vi "Vision Research Phantom Series PhFile PhGetOpenCineName.vi"(4 "Options":u32(ring) items=["0", "OFN_MULTISELECT"], 5 "Error In (no error)":errorcluster) -> (15 "szFileName":path, 18 "Success":bool, 19 "Error Out":errorcluster)   [LabVIEW 2013, in "VRI.lvlib"]
doc: "PhFile.dll\n\nPhGetOpenCineName\nBOOL PhGetOpenCineName(PSTR szFileName, UINT Options);\n\nParameters Description\nszFileName (out) Name of the file selected from the dialog box.\nOptions(in) Options available:\n 0 – The user can select only one file name.\n OFN_MULTISELECT – The user can select one or more file names.\nReturn TRUE - The operation has succeeded. The user ended the dialog with OK.\n FALSE - The operation has been canceled. The user ended the dialog with CANCEL.\nComments This function displays a dialog box, for selecting one existing cine file.\n The file name is returned in the parameter.\n\nWritten by:\nBLOOMY CONTROLS, INC\nWINDSOR, CT 06095, USA\n860-298-9925\nwww.bloomy.com\nV1.0.0\nMay, 2004"
uses:
  VRI.lvlib
  Phantom DLLs/PhFile.dll
panel:
  # "For instructions on the use of this VI, press Ctrl+H to display the help window and move the mouse over the icon, controls, and indicators"
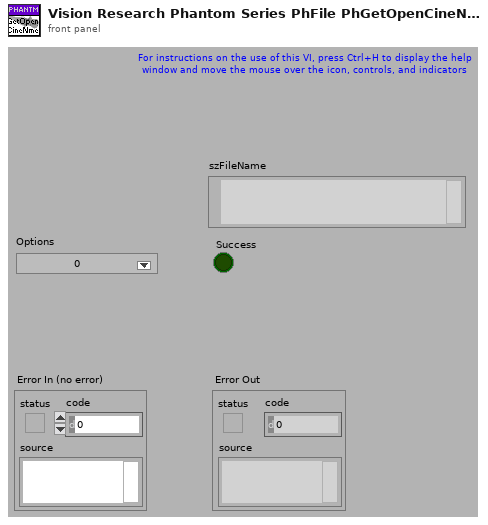
[diagram p1: front panel]
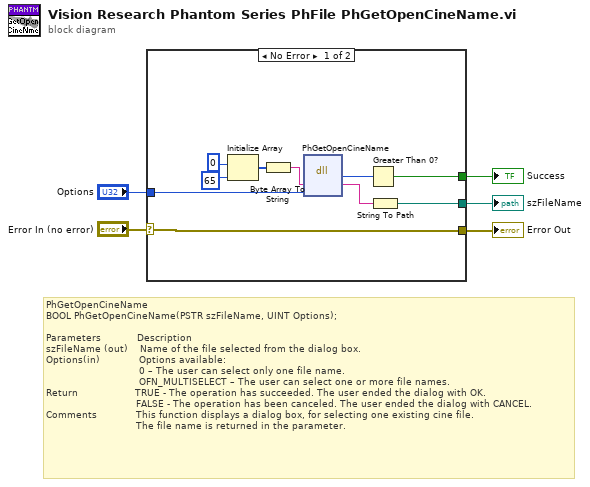
[diagram p0: block diagram]
diagram:
  # "PhGetOpenCineName\nBOOL PhGetOpenCineName(PSTR szFileName, UINT Options);\n\nParameters            Description\nszFileName (out)    Name of the file selected from the dialog box.\nOptions(in)             Options available:\n                               0 – The user can select only one file name.\n                               OFN_MULTISELECT – The user can select one or more file names.\nReturn                   TRUE - The operation has succeeded. The user ended the dialog with OK.\n                              FALSE - The operation has been canceled. The user ended the dialog with CANCEL.\nComments             This function displays a dialog box, for selecting one existing cine file.\n                              The file name is returned in the parameter."
  n1 = case shown="No Error" "Error In (no error)" {
    selector: "Error In (no error)" -> [w15 w16]
    tunnel: [w15 w16] -> w4
    tunnel: [w14 _] -> w3
    tunnel: [w13 _] -> w1
    tunnel: "Options" -> [w12 _]
    frame No Error {
      n2 = Initialize Array(u8 0, 65 ("dimension size")) -> (w9:u8[])
      n3 = Byte Array To String(unsigned byte array=w9) -> (string=w7:string)
      n4 = dll-call lib="C:/Projects/SDK/32-bit/Vision Research Phantom Series Labview Driver/Phantom DLLs/PhFile.dll" fn="PhGetOpenCineName"("szFileName"=w7, "Options"=w12) -> (w11:u8, "szFileName"=w10:string)  [unwired: 4 in, 2 out]
      n5 = Greater Than 0?(x=w11) -> (x > 0?=w14:bool)
      n6 = String To Path(string=w10) -> (path=w13:path)
    }
    frame Error {
    }
  }
  "Error Out" <- w4
  "Success" <- w3
  "szFileName" <- w1
